vi "FYP_VI_MIDI_OutMsg.vi"(5 "dwMsg dataIn":i32, 7 "midiOut hmo":i32) -> (0 "midiOutShortMsg Error Code":i32, 3 "midiOut handle":i32)   [LabVIEW 2013]
uses:
  winmm.dll
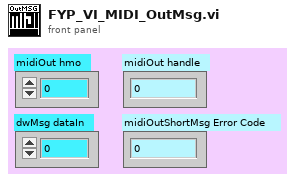
[diagram p1: front panel]
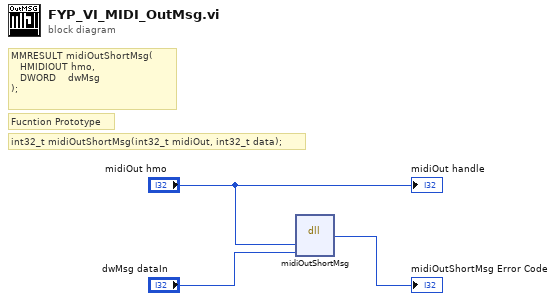
[diagram p0: block diagram]
diagram:
  # "Fucntion Prototype"
  # "int32_t midiOutShortMsg(int32_t midiOut, int32_t data);"
  # "MMRESULT midiOutShortMsg(\n   HMIDIOUT hmo,\n   DWORD    dwMsg\n);"
  n1 = dll-call lib="winmm.dll" fn="midiOutShortMsg"("midiOut"="midiOut hmo", "data"="dwMsg dataIn") -> ("return type"=→"midiOutShortMsg Error Code":i32)  [unwired: 5 in, 2 out]
  "midiOut handle" <- "midiOut hmo"
